vi "XY Graph Update Plot.vi"(4 "Y Array":dbl[](array[numeric]), 6 "X Array":dbl[](array[numeric]), 7 "New Plot Name (Default: unchanged)":string, 8 "Error In":errorcluster, 9 "Plot":cluster{"X Array":dbl[], "Y Array":dbl[]}, 10 "Plot Idx":i32, 11 "XY Graph refnum":T1) -> (0 "Error Out":errorcluster)   [LabVIEW 2021, in "XY Graph Add-Ons.lvlib"]
doc: "Update the Plot whose index is provided using either the Plot structure (first) or, if empty, the X and Y arrays.\nIf all are empty, then an empty plot is replacing the selected one."
uses:
  XY Graph Refnum.ctl
  XY Graph Add-Ons.lvlib
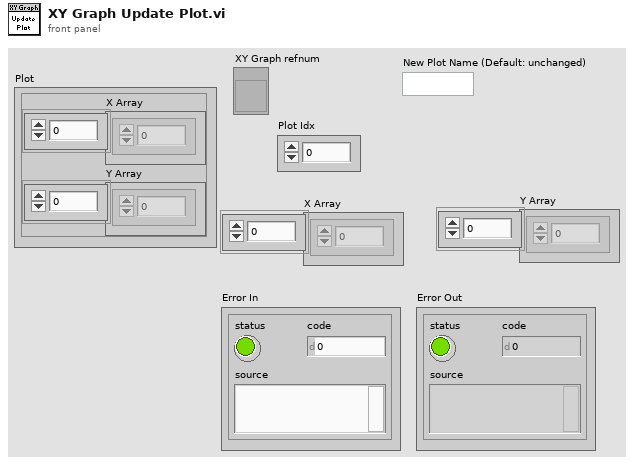
[diagram p1: front panel]
types:
  T1 = typedef "XY Graph Add-Ons.lvlib/XY Graph Refnum.ctl" = refnum<vi>
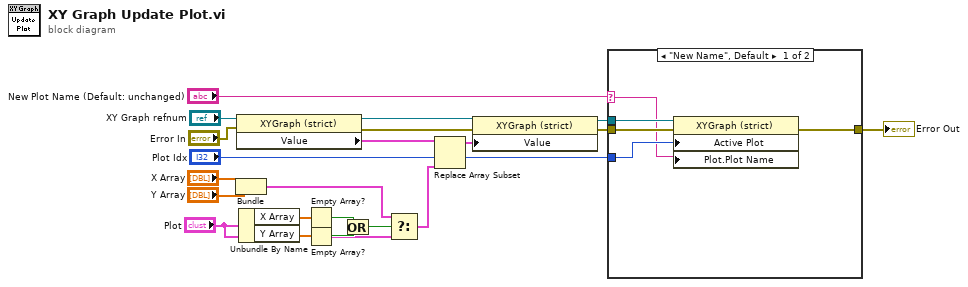
[diagram p0: block diagram]
diagram:
  n1 = Bundle("X Array"="X Array", "Y Array"="Y Array") -> (w8:cluster{"X Array":dbl[], "Y Array":dbl[]})  [unwired: 1 in]
  n2 = property class="XYGraph (strict)"(reference="XY Graph refnum", error in="Error In") -> (reference out=w17:T1, error out=w16:errorcluster, "Value"=w20:cluster{"X Array":dbl[], "Y Array":dbl[]}[])
  n3 = Unbundle By Name("Plot") -> ("X Array"=w13:dbl[], "Y Array"=w12:dbl[])
  n4 = Empty Array?(array=w13) -> (empty?=w11:bool)
  n5 = Empty Array?(array=w12) -> (empty?=w10:bool)
  n6 = Or(x=w11, y=w10) -> (x .or. y?=w9:bool)
  n7 = Select(t=w8, s=w9, f="Plot") -> (s? t:f=w6:cluster{"X Array":dbl[], "Y Array":dbl[]})
  n8 = Replace Array Subset(array=w20, new element=w6, index="Plot Idx") -> (w15:cluster{"X Array":dbl[], "Y Array":dbl[]}[])
  n9 = property class="XYGraph (strict)"(reference=w17, error in=w16, "Value"=w15) -> (reference out=w2:T1, error out=w4:errorcluster)
  n10 = case shown="\"New Name\", Default" "New Plot Name (Default: unchanged)" {
    selector: "New Plot Name (Default: unchanged)" -> [w23 _]
    tunnel: w4 -> [w25 w27]
    tunnel: [w22 w27] -> w3
    tunnel: w2 -> [w26 _]
    tunnel: "Plot Idx" -> [w24 _]
    frame "New Name", Default {
      n11 = property class="XYGraph (strict)"(reference=w26, error in=w25, "Active Plot"=w24, "Plot.Plot Name"=w23) -> (error out=w22:errorcluster)  [unwired: 1 out]
    }
    frame "" {
      # "unchanged"
    }
  }
  "Error Out" <- w3
